vi "RequestApproval.vi"(8 "error in (no error)":errorcluster, 10 "calibration_id":i32, 11 "ByteGSAPIBase in":refnum<class "ByteGSAPIBase.lvclass">) -> (0 "error out":errorcluster, 2 "controls":T1(array[cluster]), 3 "ByteGSAPIBase out":refnum<class "ByteGSAPIBase.lvclass">)   [LabVIEW 2019, in "ByteGSWebAPI.lvlib" / "ByteGSAPIBase.lvclass"]
uses:
  ByteGSAPIBase.lvclass
  <vilib>/Bytelabs/ByteREST/ByteRESTClass/ByteRESTBase/HTTP/Status_Code.ctl
  ApprovalOutputCluster.ctl
  ByteGSAPIBase.lvclass/ByteGSAPIBase.ctl
  <vilib>/Bytelabs/ByteREST/ByteRESTClass/ByteRESTBase/RESTBase.lvclass
panel:
  in  "send notification":bool
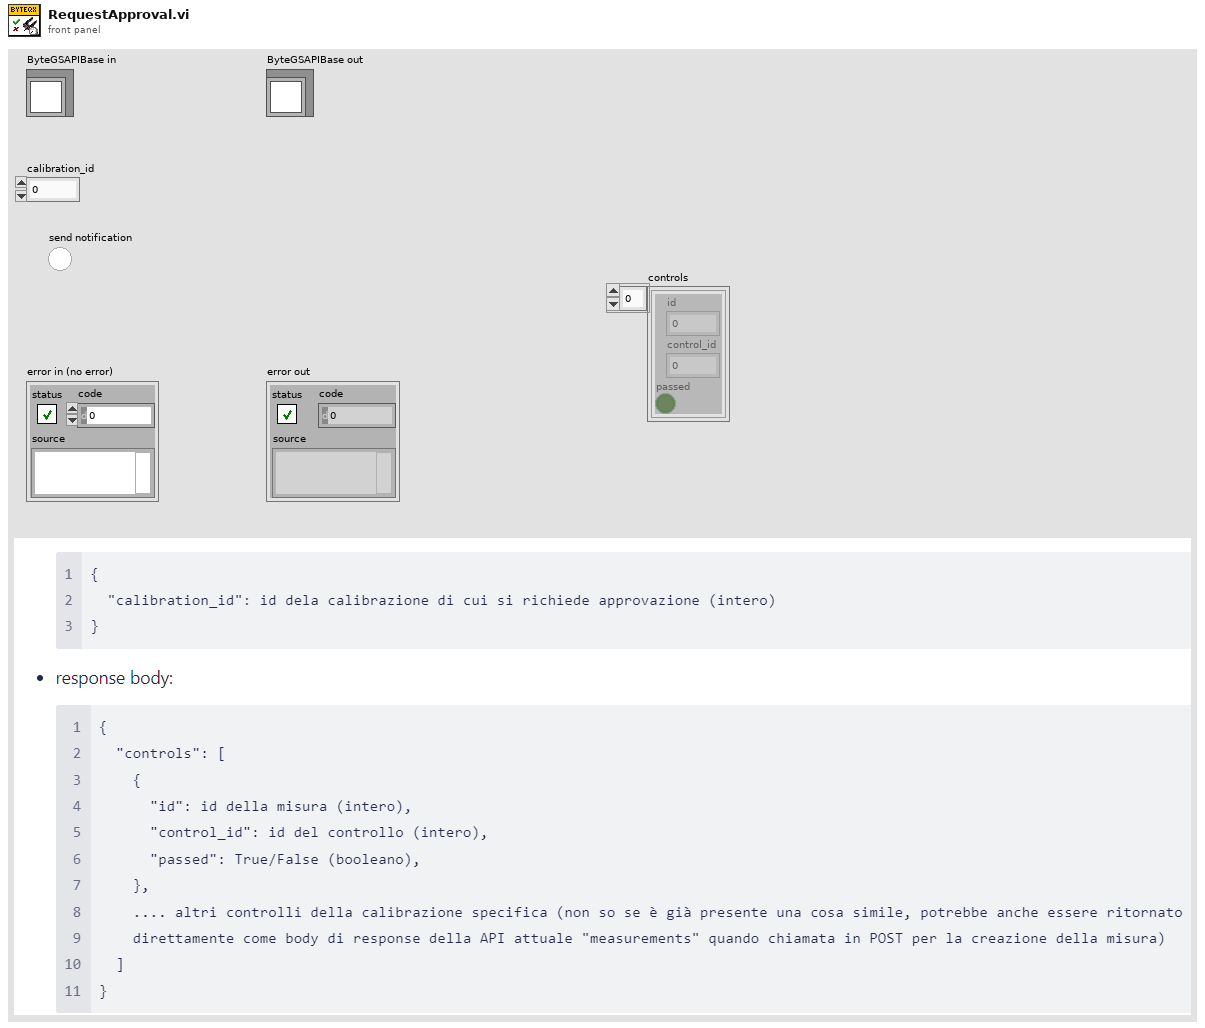
[diagram p1: front panel]
types:
  T1 = cluster{"id":u32, "control_id":u32, "passed":bool}[]
  T2 = typedef "ByteGSWebAPI.lvlib/ByteGSAPIBase.lvclass/ApprovalOutputCluster.ctl" = cluster{"controls":cluster{"id":u32, "control_id":u32, "passed":bool}[]}
  T3 = cluster{"calibration_id":i32, "notification_active":bool}
  T4 = typedef "ByteREST.lvlib/RESTBase.lvclass/Status_Code.ctl" = u16
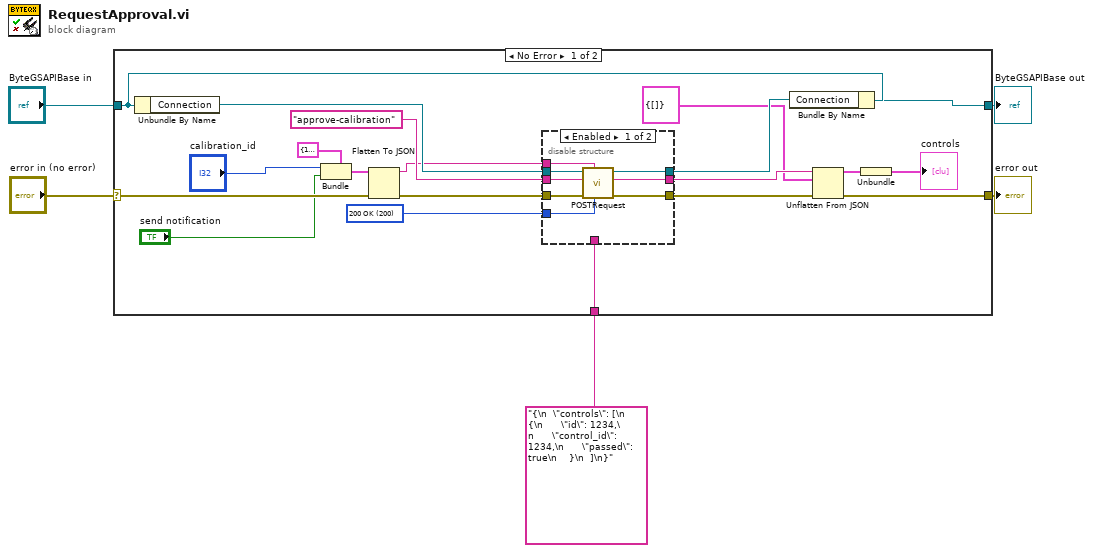
[diagram p0: block diagram]
diagram:
  n1 = case shown="No Error" "error in (no error)" {
    selector: "error in (no error)" -> [w20 w36]
    tunnel: [w14 w36] -> w4
    tunnel: [w23 w35] -> w2
    tunnel: "ByteGSAPIBase in" -> [w25 w35]
    tunnel: "{\n  \"controls\": [\n    {\n      \"id\": 1234,\n      \"control_id\": 1234,\n      \"passed\": true\n    }\n  ]\n}" -> [w10 _]
    frame No Error {
      w17 = T4 200 items=["200 OK"=200, "201 Created"=201, "400 Bad Request"=400, "401 Unauthorized"=401, "403 Forbidden"=403, "404 Not Found"=404, "405 Method Not Allowed"=405, "406 Not Acceptable"=406, "500 Internal Server Error"=500] ("expected response")
      n2 = Unbundle By Name(w25) -> ("Connection"=w24:refnum<class "RESTBase.lvclass">)
      n3 = Bundle(cluster=T3 {"calibration_id"=1234, "notification_active"=FALSE}, "calibration_id"="calibration_id", "notification_active"="send notification") -> (w11:T3)
      n4 = Flatten To JSON(anything=w11, error in (no error)=w20) -> (JSON string=w15:string, 11:w16:errorcluster)  [unwired: 1 in]
      n5 = disable-structure shown="Enabled" {
        disable-tunnel: w24 -> [w33 _]
        disable-tunnel: [w32 _] -> w22
        disable-tunnel: "approve-calibration" ("Request") -> [w31 _]
        disable-tunnel: [w30 w34] -> w19
        disable-tunnel: [w29 _] -> w18
        disable-tunnel: w17 -> [w28 _]
        disable-tunnel: w16 -> [w27 _]
        disable-tunnel: w15 -> [w26 _]
        disable-tunnel: w10 -> [_ w34]
        frame Enabled {
          n6 = call-dynamic "POSTRequest.vi"("expected response"=w28, "Body in"=w26, "error in (no error)"=w27, "Request"=w31, "ByteRESTBase in"=w33) -> ("error out"=w29:errorcluster, "Body"=w30:string, "ByteRESTBase out"=w32:refnum<class "RESTBase.lvclass">)  [unwired: 3 in, 1 out]
        }
        frame Disabled {
        }
      }
      n7 = Bundle By Name(cluster=w25, "Connection"=w22) -> (w23:refnum<class "ByteGSAPIBase.lvclass">)
      n8 = Unflatten From JSON(JSON string=w19, type and defaults=T2 {"controls"=[]}, error in (no error)=w18) -> (value=w8:T2, error out=w14:errorcluster)  [unwired: 4 in]
      n9 = Unbundle(w8) -> ("controls"=→"controls":T1)
    }
    frame Error {
    }
  }
  "error out" <- w4
  "ByteGSAPIBase out" <- w2
